vi "GalvoGotoPos.vi"(0 "Galvo-resource in":T1, 1 "Zwischenbild (m/bit)":dbl=9.321e-09, 2 "Pos":cluster{"x":dbl, "y":dbl}, 3 "error in":errorcluster) -> (5 "Galvo-resource out":T1, 6 "error out":errorcluster)   [LabVIEW 2011]
uses:
  SIAM/SIAM_command.ctl
  SIAM/SIAM-send.ctl
  <vilib>/DAQmx/write.llb/DAQmx Write (Analog 2D I16 NChan NSamp).vi
  <vilib>/DAQmx/create/channels.llb/DAQmx Create Channel (AO-Voltage-Basic).vi
  <vilib>/DAQmx/miscellaneous.llb/DAQmx Fill In Error Info.vi
  National Instruments/LabVIEW 2011/resource/objmgr/daqmx.rc
panel:
  out "write":string
  out "read buffer":string
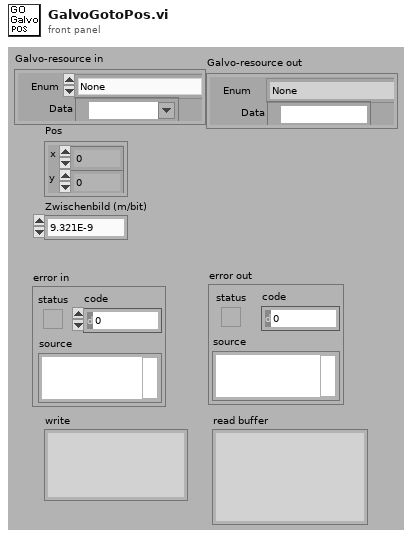
[diagram p1: front panel]
types:
  T1 = cluster{"Enum":enum16{"None", "DSP-on serial port", "Analog out", "SIAM-withDSiam"}, "Data":refnum<k21>}
  T2 = enum16{"None", "DSP-on serial port", "Analog out", "SIAM-withDSiam"}
  T3 = enum16{"Com", "Digital", "Analog", "GalvoX", "GalvoY", "GalvoCCD", "Free1", "Free2", "Free3", "Loop", "SMoveTime", "Image1X", "Image1Y", "Image2X", "Image2Y"}
  T4 = typedef "SIAM_command.ctl" = u32
  T5 = cluster{"Delay 10µs":u32, "command":T4, "P0":i32, "P1":i32, "P2":i32, "P3":i32, "P4":i32, "P5-ticket":i32}
  T6 = typedef "SIAM-send.ctl" = enum16{"validID", "storeID", "enable", "rundirect", "sendlist", "run", "stop", "readRegister", "sendValue", "storeStatus"}
  T7 = enum16{"Ch0", "Ch1", "x-Galvo", "y-Galvo", "z-Focus"}[]
  T8 = cluster{"Delay 10µs":u32, "command":T4, "P0":i32, "P1":i32, "P2":i32, "P3":i32, "P4":i32, "P5-ticket":i32}[]
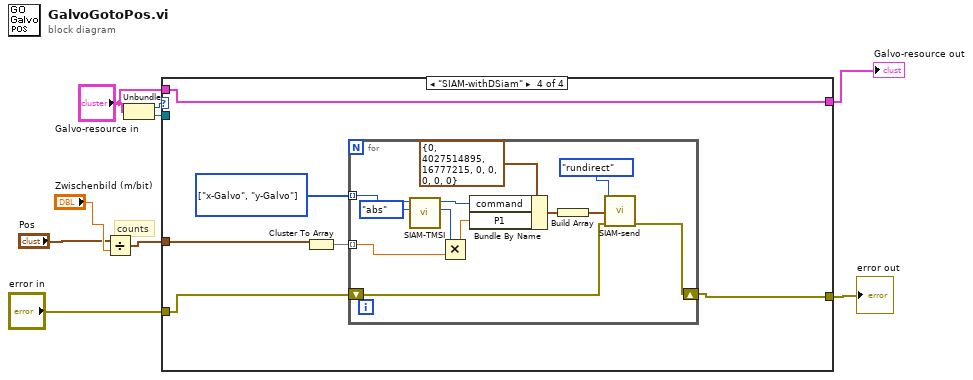
[diagram p0: block diagram]
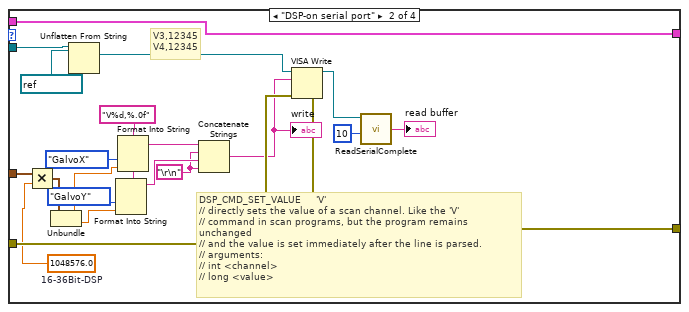
[diagram p3: hidden frame]
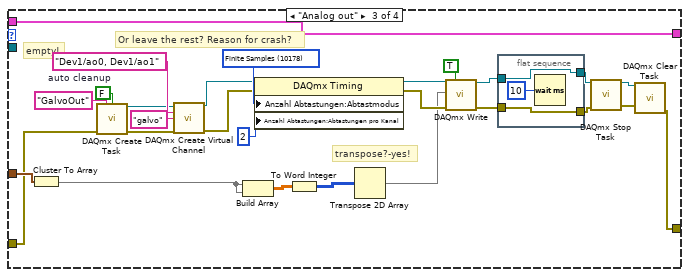
[diagram p4: hidden frame]
diagram:
  # "counts"
  n1 = Divide(x="Pos", y="Zwischenbild (m/bit)") -> (x/y=w4:cluster{"x":dbl, "y":dbl})
  n2 = Unbundle("Galvo-resource in") -> ("Enum"=w7:T2, "Data"=w6:refnum<k21>)
  n3 = case shown="\"SIAM-withDSiam\"" w7 {
    tunnel: "error in" -> [w11 w32 w41 w64]
    tunnel: [w11 w31 w36 w63] -> w8
    tunnel: w6 -> [_ w30 _ _]
    tunnel: w4 -> [_ w20 w54 w67]
    tunnel: [w10 w12 w33 w68] -> w2
    tunnel: "Galvo-resource in" -> [w10 w12 w33 w68]
    frame "None", Default {
    }
    frame "DSP-on serial port" {
      w13 = 1048576.0  # 16-36Bit-DSP
      w22 = "\r\n"
      w25 = "V%d,%.0f" ("Format String")
      # "V3,12345\nV4,12345"
      # "DSP_CMD_SET_VALUE     'V'    \n// directly sets the value of a scan channel. Like the 'V' \n// command in scan programs, but the program remains unchanged\n// and the value is set immediately after the line is parsed.\n// arguments:\n// int <channel>\n// long <value>"
      n4 = Multiply(x=w20, y=w13) -> (x*y=w19:cluster{"x":dbl, "y":dbl})
      n5 = Unbundle(w19) -> ("x"=w18:dbl, "y"=w17:dbl)
      n6 = Unflatten From String(type=refnum<visa-resource-name> "COM1" ("DSP resource name out"), binary string=w30) -> (value=w28:refnum<visa-resource-name>)  [unwired: 1 in, 4 out]
      n7 = Format Into String(format string=w25, T3."GalvoY" ("Kanal"), w17) -> (resulting string=w23:string)  [unwired: 2 in, 1 out]
      n8 = Format Into String(format string=w25, T3."GalvoX" ("Kanal"), w18) -> (resulting string=w24:string)  [unwired: 2 in, 1 out]
      n9 = Concatenate Strings(w24, w22, w23, w22) -> (w21:string)
      "write" <- w21
      n10 = VISA Write(VISA resource name=w28, write buffer=w21, error in (no error)=w32) -> (VISA resource name out=w16:refnum<visa-resource-name>, error out=w31:errorcluster)  [unwired: 1 out]
      n11 = call "ReadSerialComplete.vi"("milliseconds to wait"=u32 10, "duplicate VISA resource name"=w16) -> ("read buffer"=→"read buffer":string)  [unwired: 2 in, 2 out]
    }
    frame "Analog out" {
      w44 = FALSE  # auto cleanup
      w51 = 10178 items=["Finite Samples"=10178, "Continuous Samples"=10123, "Hardware Timed Single Point"=12522] ("SampQuant.SampMode")
      # "empty!"
      # "transpose?-yes!"
      # "Or leave the rest? Reason for crash?"
      n12 = Cluster To Array(cluster=w54) -> (array=w53:dbl[])
      n13 = call <vilib>:"DAQmx Create Task.vi"("new task name"="GalvoOut", "auto cleanup"=w44, "error in"=w41) -> ("task out"=w45:refnum<k21>, "error out"=w46:errorcluster)  [unwired: 2 in, 9 out]
      n14 = call-poly <vilib>:"DAQmx Create Virtual Channel.vi"("task in"=w45, "physical channels"="Dev1/ao0, Dev1/ao1" ("names out"), "name to assign"="galvo", "error in"=w46) -> ("task out"=w43:refnum<k21>, "error out"=w42:errorcluster)  [unwired: 5 in, 5 out]
      n15 = Build Array(w53, w53) -> (w55:dbl[][])
      n16 = property class="DAQmx Timing"(reference=w43, error in=w42, "Anzahl Abtastungen:Abtastmodus"=w51, "Anzahl Abtastungen:Abtastungen pro Kanal"=2 ("samples per channel")) -> (reference out=w58:refnum<k21>, error out=w57:errorcluster)
      n17 = To Word Integer(number=w55) -> (16bit integer=w56:i16[][])
      n18 = Transpose 2D Array(2D array=w56) -> (transposed array=w52:i16[][])
      n19 = call-poly <vilib>:"DAQmx Write.vi"("task/channels in"=w58, "auto start"=TRUE, "data"=w52, "error in"=w57) -> ("task out"=w35:refnum<k21>, "error out"=w40:errorcluster)  [unwired: 10 out]
      n20 = flat-sequence {
        tunnel: w40 -> [w61]
        tunnel: [w61] -> w37
        tunnel: w35 -> [w60]
        tunnel: [w60] -> w34
        frame #0 {
          n21 = Wait (ms)(milliseconds to wait=u32 10) -> ()  [unwired: 1 out]
        }
      }
      n22 = call <vilib>:"DAQmx Stop Task.vi"("task/channels in"=w34, "error in"=w37) -> ("task out"=w38:refnum<k21>, "error out"=w39:errorcluster)  [unwired: 12 out]
      n23 = call <vilib>:"DAQmx Clear Task.vi"("task in"=w38, "error in"=w39) -> ("error out"=w36:errorcluster)  [unwired: 13 out]
    }
    frame "SIAM-withDSiam" {
      w66 = T7 [enum."x-Galvo", enum."y-Galvo"] items=["Ch0", "Ch1", "x-Galvo", "y-Galvo", "z-Focus"]
      n24 = Cluster To Array(cluster=w67) -> (array=w65:dbl[])
      n25 = for {
        tunnel: w66 -> [w75] mode=indexing
        tunnel: w65 -> [w72] mode=indexing
        shift-right: [w76] -> w63
        shift-left: w64 -> [w77]
        n26 = call "SIAM-TMSI.vi"("Type"=enum8{"acc", "vel", "abs", "offset"}."abs", "Motor"=w75) -> ("Resolution-Factor"=w71:i32, "command"=w73:T4)  [unwired: 6 in, 2 out]
        n27 = Multiply(x=w71, y=w72) -> (x*y=w70:dbl)
        n28 = Bundle By Name(cluster=T5 {"Delay 10µs"=0, "command"=4027514895, "P0"=16777215, "P1"=0, "P2"=0, "P3"=0, "P4"=0, "P5-ticket"=0} ("Cluster"), "command"=w73, "P1"=w70) -> (w79:T5)
        n29 = Build Array(w79) -> (w78:T8)
        n30 = call "SIAM-send.vi"("error in (no error)"=w77, "Script"=w78, "command"=SIAM-send."rundirect") -> ("error out"=w76:errorcluster)  [unwired: 7 in, 1 out]
      }
    }
  }
  "error out" <- w8
  "Galvo-resource out" <- w2
